vi "MicroPulse - RF slots decoder.vi"(1 "byte array":u8[](array[numeric]) format="%.0b") -> (0 "RF Slot status":string)   [LabVIEW 2026, in "MicroPulse_Driver.lvlib"]
uses:
  MicroPulse_Driver.lvlib
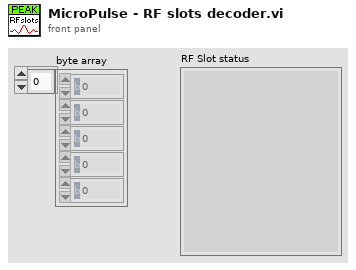
[diagram p1: front panel]
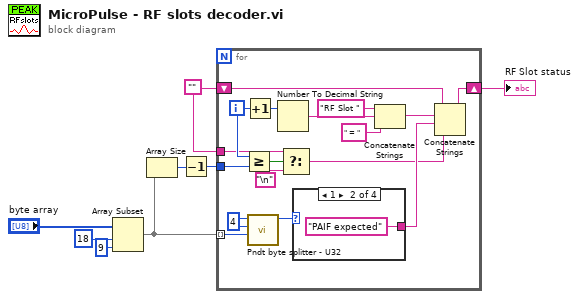
[diagram p0: block diagram]
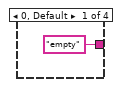
[diagram p2: hidden frame]
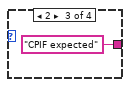
[diagram p3: hidden frame]
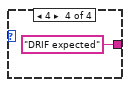
[diagram p4: hidden frame]
diagram:
  w1 = ""
  n1 = Array Subset(array="byte array", index=18, length=9) -> (w4:u8[])
  n2 = Array Size(array=w4) -> (size(s)=w3:i32)
  n3 = Decrement(x=w3) -> (x-1=w2:i32)
  n4 = for {
    tunnel: w4 -> [w24] mode=indexing
    shift-right: [w15] -> w5
    shift-left: w1 -> [w16]
    tunnel: w2 -> [w13]
    tunnel: w1 -> [w10]
    i -> [w14]
    w25 = i16 4 ("y")
    n5 = Greater Or Equal?(x=w14, y=w13) -> (x >= y?=w12:bool)
    n6 = Increment(x=w14) -> (x+1=w18:i32)
    n7 = call "Pndt byte splitter - U32.vi"("byte U32"=w24, "mask size"=w25, "shift right"=w25) -> ("hi"=w23:u32)  [unwired: 7 in, 1 out]
    n8 = Number To Decimal String(number=w18) -> (decimal integer string=w19:string)  [unwired: 1 in]
    n9 = Select(t=w10, s=w12, f="\n") -> (s? t:f=w9:string)
    n10 = case shown="1" w23 {
      tunnel: ["empty" "PAIF expected" "CPIF expected" "DRIF expected"] -> w22
      frame 0, Default {
      }
      frame 1 {
      }
      frame 2 {
      }
      frame 4 {
      }
    }
    n11 = Concatenate Strings("RF Slot ", w19, " = ") -> (w20:string)
    n12 = Concatenate Strings(w16, w20, w22, w9) -> (w15:string)
  }
  "RF Slot status" <- w5
